vi "Calibrate_ESC.vi"(1 "Min Duty Cycle (%)":dbl=5.0 format="%#_13g", 2 "Max Duty Cycle (%)":dbl=10.0 format="%#_13g") -> ()   [LabVIEW 2015]
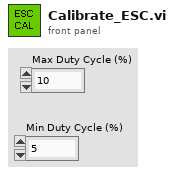
[diagram p1: front panel]
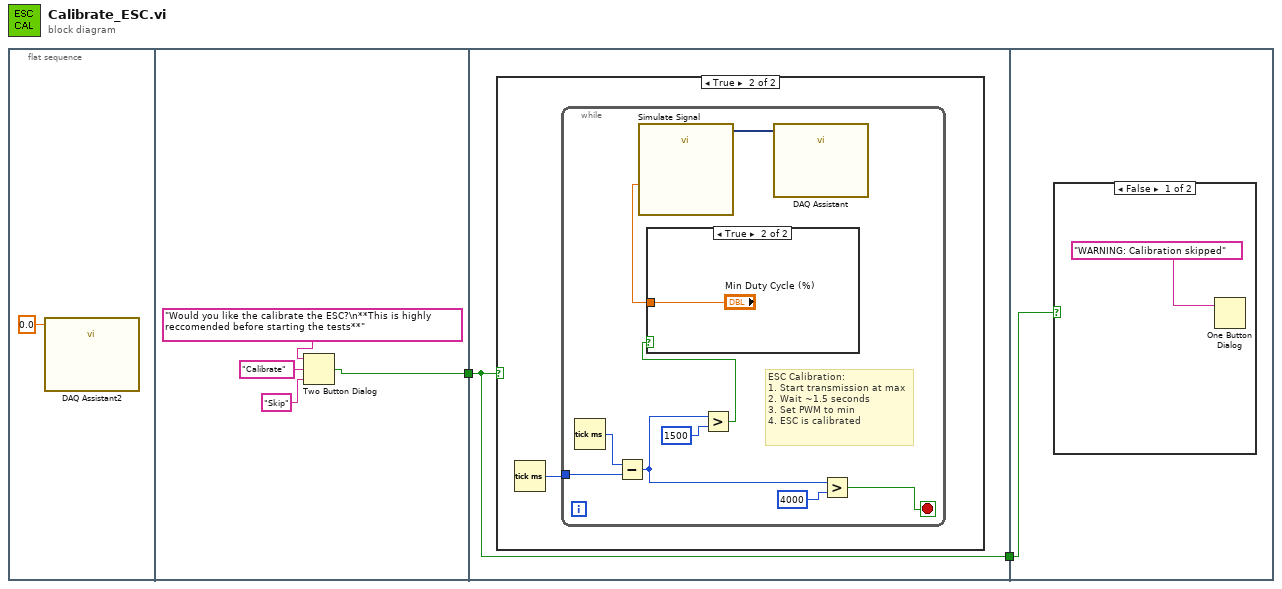
[diagram p0: block diagram]
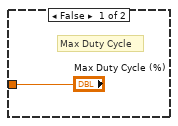
[diagram p3: hidden frame]
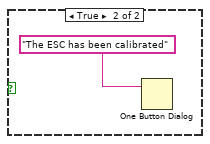
[diagram p4: hidden frame]
diagram:
  n1 = flat-sequence {
    tunnel: [w4] -> w2
    tunnel: w2 -> [w8]
    tunnel: [w8] -> w1
    tunnel: w1 -> [w21]
    frame #0 {
      n2 = call "DAQ Assistant2"("data"=0.0) -> ()  [unwired: 17 in, 2 out]
    }
    frame #1 {
      n3 = Two Button Dialog(message="Would you like the calibrate the ESC?\n**This is highly reccomended before starting the tests**", 1:"Skip" ("F button name (\"Cancel\")"), 2:"Calibrate" ("T button name (\"OK\")")) -> (T button?=w4:bool)
    }
    frame #2 {
      n4 = case shown="True" w8 {
        frame False {
          # "Do not Calibrate if false."
        }
        frame True {
          n5 = Tick Count (ms)() -> (millisecond timer value=w9:u32)
          n6 = while {
            tunnel: w9 -> [w17]
            stop <- w10 stop-if-true
            # "ESC Calibration:\n1. Start transmission at max\n2. Wait ~1.5 seconds\n3. Set PWM to min\n4. ESC is calibrated"
            n7 = Tick Count (ms)() -> (millisecond timer value=w15:u32)
            n8 = Subtract(x=w15, y=w17) -> (x-y=w12:u32)
            n9 = Greater?(x=w12, y=u32 1500) -> (0:w13:bool)
            n10 = case shown="True" w13 {
              tunnel: ["Max Duty Cycle (%)" "Min Duty Cycle (%)"] -> w14
              frame False {
                # "Max Duty Cycle"
              }
              frame True {
              }
            }
            n11 = call "Simulate Signal"("Duty Cycle (%)"=w14) -> ("Square"=w18:dynamicdata)  [unwired: 13 in, 1 out]
            n12 = call "DAQ Assistant"("data"=w18) -> ()  [unwired: 16 in, 3 out]
            n13 = Greater?(x=w12, y=u32 4000) -> (0:w10:bool)
          }
        }
      }
    }
    frame #3 {
      n14 = case shown="False" w21 {
        frame False {
          n15 = One Button Dialog(message="WARNING: Calibration skipped") -> ()  [unwired: 1 in, 1 out]
        }
        frame True {
          n16 = One Button Dialog(message="The ESC has been calibrated") -> ()  [unwired: 1 in, 1 out]
        }
      }
    }
  }
